vi "Scan_from_string.vi"() -> ()   [LabVIEW 2019]
panel:
  out "Place":string
  out "Age":i32
  out "Profession":string
  out "Name":string
  in  "String":string="I am Tejaswini , I am going to be an Engineer soon . My age is 20 and I live in Nagpur ."
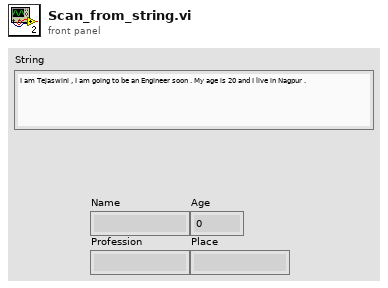
[diagram p1: front panel]
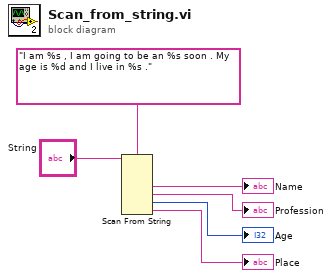
[diagram p0: block diagram]
diagram:
  n1 = Scan From String(format string="I am %s , I am going to be an %s soon . My age is %d and I live in %s .", input string="String") -> (output 1=→"Name":string, output 2=→"Profession":string, output 3=→"Age":i32, output 4=→"Place":string)  [unwired: 6 in, 3 out]
